vi "UartRxRead.vi"(8 "error in (no error)":errorcluster caption="错误输入（无错误）", 10 "length":i32=256, 11 "handle":u64) -> (0 "error out":errorcluster caption="错误输出", 1 "rgRX":u8[](array[numeric]), 2 "function return":i32, 3 "handle out":u64, 4 "rxcount out":i32)   [LabVIEW 2018]
doc: "Uart read data"
uses:
  InstrumentsPlayground.lvlib
panel:
  out "fParity out":i32
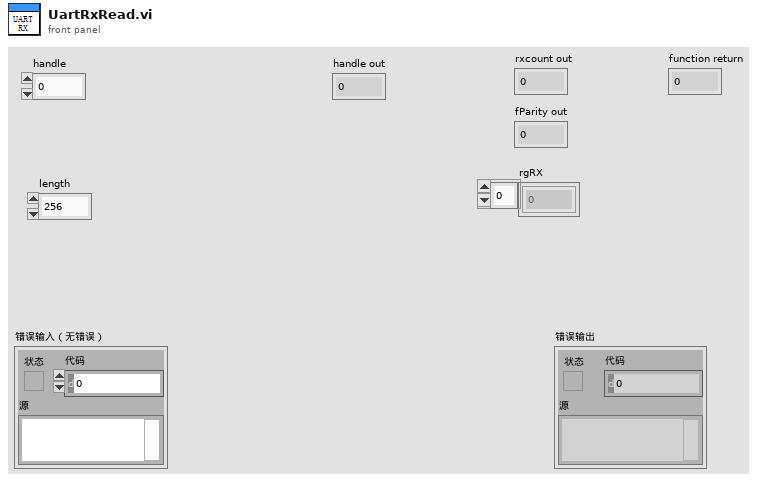
[diagram p1: front panel]
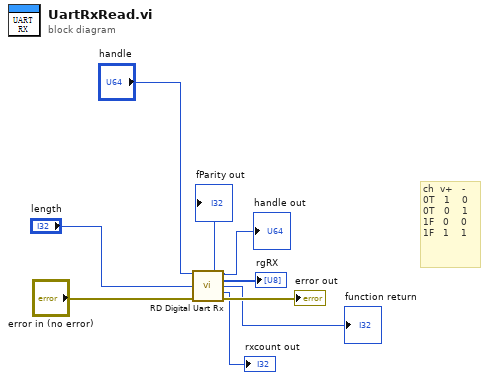
[diagram p0: block diagram]
diagram:
  # "ch  v+   -\n0T   1    0\n0T   0    1\n1F   0    0\n1F   1    1"
  n1 = call "RD Digital Uart Rx.vi"("handle"="handle", "length"="length", "error in (no error)"="error in (no error)") -> ("fParity out"=→"fParity out":i32, "handle out"=→"handle out":u64, "rgRX"=→"rgRX":u8[], "function return"=→"function return":i32, "rxcount out"=→"rxcount out":i32, "error out"=→"error out":errorcluster)  [unwired: 7 in]
